vi "BRig_dataLC_Cue_PreR_Prob_l1.vi"() -> (2 "output_Cue_PreR_Prob":i32)   [LabVIEW 2014]
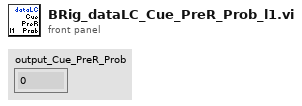
[diagram p1: front panel]
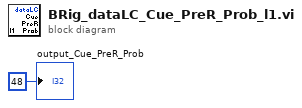
[diagram p0: block diagram]
diagram:
  "output_Cue_PreR_Prob" <- 48 ("output_iBlock")
